vi "Post-Dig Hook.vi"(8 "Error In":errorcluster) -> (0 "Error Out":errorcluster)   [LabVIEW 2018, in "Tests.lvlib" / "Toolkit.lvlib" / "Integration.lvlib"]
uses:
  Integration.lvlib
  Support/Dig Target.vi
  src/Toolkit/Toolkit.lvlib
  <vilib>/addons/_JKI Toolkits/Caraya/classes/Test/Test.lvclass
  Tests.lvlib
  <vilib>/addons/_JKI Toolkits/Caraya/classes/Assert/Assert.lvclass
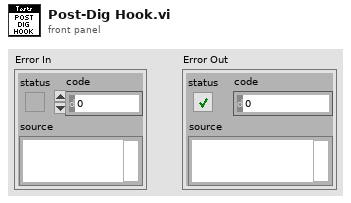
[diagram p1: front panel]
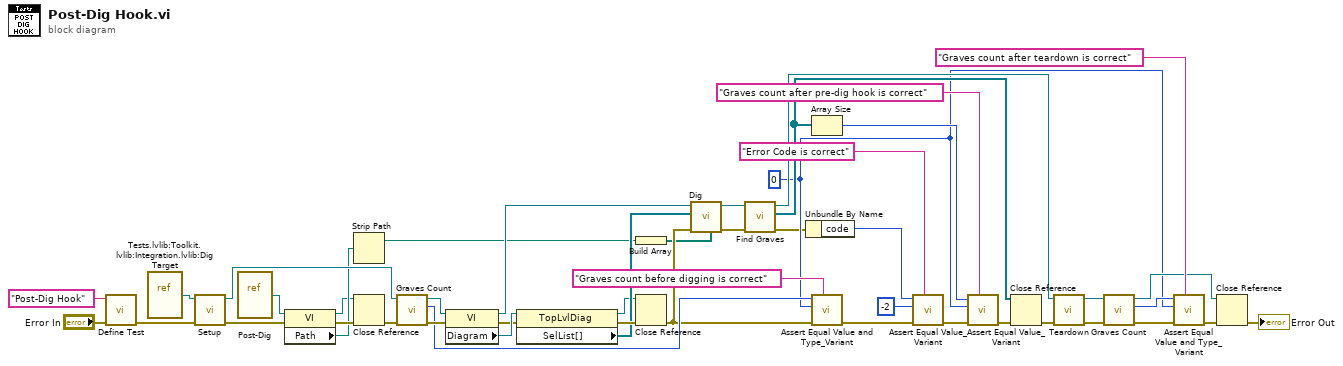
[diagram p0: block diagram]
diagram:
  w6 = 0 ("size(s)")
  n1 = call <vilib>:"Define Test.vi"("error in (no error)"="Error In", "Label (VI Title)"="Post-Dig Hook") -> ("error out"=w26:errorcluster)  [unwired: 9 in]
  n2 = vi-ref "Tests.lvlib:Toolkit.lvlib:Integration.lvlib:Dig Target.vi"() -> (w2:refnum<vi>)
  n3 = call "Setup.vi"("Error In"=w26, "VI In"=w2) -> ("Error Out"=w12:errorcluster, "VI Out"=w28:refnum<vi>)  [unwired: 8 in]
  n4 = vi-ref "Post-Dig.vi"() -> (w13:refnum<vi>)
  n5 = property class="VI"(reference=w13, error in=w12) -> (reference out=w7:refnum<vi>, error out=w11:errorcluster, "Path"=w10:path)
  n6 = Strip Path(path=w10) -> (stripped path=w9:path)  [unwired: 1 out]
  n7 = Close Reference(reference=w7, error in (no error)=w11) -> (error out=w8:errorcluster)
  n8 = call "Graves Count.vi"("Error In"=w8, "Test Target In"=w28) -> ("Error Out"=w23:errorcluster, "Graves Count"=w22:i32, "Test Target Out"=w27:refnum<vi>)  [unwired: 7 in]
  n9 = property class="VI"(reference=w27, error in=w23) -> (reference out=w44:refnum<vi>, error out=w46:errorcluster, "Diagram"=w47:refnum<vi>)
  n10 = property class="TopLvlDiag"(reference=w47, error in=w46) -> (reference out=w37:refnum<vi>, error out=w45:errorcluster, "SelList[]"=w43:refnum<vi>[])
  n11 = Build Array(w9) -> (w1:path[])
  n12 = Close Reference(reference=w37, error in (no error)=w45) -> (error out=w19:errorcluster)
  n13 = call "Dig.vi"("Hooks Search Path"=w1, "Error In"=w19, "Selection List[]"=w43, "VI In"=w44) -> ("Error Out"=w42:errorcluster, "VI Out"=w29:refnum<vi>)  [unwired: 6 in]
  n14 = call "Find Graves.vi"("Error In"=w42, "VI In"=w29) -> ("Error Out"=w5:errorcluster, "Graves"=w31:refnum<vi>[], "VI Out"=w33:refnum<vi>)  [unwired: 7 in]
  n15 = Unbundle By Name(w5) -> ("code"=w4:i32)
  n16 = Array Size(array=w31) -> (size(s)=w36:i32)
  n17 = call <vilib>:"Assert Equal Value and Type_Variant.vi"("Label"="Graves count before digging is correct", "error in (no error)"=w19, "Y"=w6, "X"=w22) -> ("error out"=w25:errorcluster)  [unwired: 7 in]
  n18 = call <vilib>:"Assert Equal Value_Variant.vi"("Label"="Error Code is correct", "error in (no error)"=w25, "Y"=-2 ("code"), "X"=w4) -> ("error out"=w39:errorcluster)  [unwired: 7 in]
  n19 = call <vilib>:"Assert Equal Value_Variant.vi"("Label"="Graves count after pre-dig hook is correct", "error in (no error)"=w39, "Y"=w6, "X"=w36) -> ("error out"=w34:errorcluster)  [unwired: 7 in]
  n20 = Close Reference(reference=w31, error in (no error)=w34) -> (error out=w30:errorcluster)
  n21 = call "Teardown.vi"("Error In"=w30, "VI In"=w33) -> ("Error Out"=w16:errorcluster, "VI Out"=w18:refnum<vi>)  [unwired: 8 in]
  n22 = call "Graves Count.vi"("Error In"=w16, "Test Target In"=w18) -> ("Error Out"=w15:errorcluster, "Graves Count"=w14:i32, "Test Target Out"=w17:refnum<vi>)  [unwired: 7 in]
  n23 = call <vilib>:"Assert Equal Value and Type_Variant.vi"("Label"="Graves count after teardown is correct", "error in (no error)"=w15, "Y"=w6, "X"=w14) -> ("error out"=w21:errorcluster)  [unwired: 7 in]
  n24 = Close Reference(reference=w17, error in (no error)=w21) -> (error out=→"Error Out":errorcluster)
